vi "ni579x Send User Command.vi"(0 "Register Bus":T3, 1 "scope":string, 5 "User Command":T1 {"User Command ID" items=["Set Clock Select"=0, "Set CLK OUT Source"=1, "DAC Sync User Start"=2, "DAC Sync User End"=3, "Enable Baseband Amp"=5, "Set Rx Attenuation Pre-LNA"=7, "Set Rx Attenuation Post-LNA"=8, "Set Tx Attenuation"=9, "Set LO Filter"=32, "Set Front End Filter"=33, "Enable LO"=34, "Set Routing Mux"=37, "Read Current Rev Lower"=240, "Read Current Rev Upper"=241, "Read Oldest Compat Rev Lower"=242, "Read Oldest Compat Rev Upper"=243, "Re-Initialize"=255]; "User Data 1" format="%x"; "User Data 0" format="%x"}, 9 "timeout":dbl=1.0, 11 "Error In":errorcluster, 12 "wait for completion?":bool=TRUE, 13 "read return values?":bool=TRUE) -> (4 "Register Bus (out)":T3, 6 "user command status":u8, 8 "user return value":u16, 10 "user command error":u8, 15 "Error Out":errorcluster)   [LabVIEW 2015, in "ni579x Config v2 Host.lvlib"]
uses:
  <instrlib>/ni579x/Config/v2/Host/ni579x Config v2 Host.lvlib
  <instrlib>/_niInstr/Register Bus/v0/Host/Public/Register Bus Session.ctl
  <instrlib>/_niInstr/Register Bus/v0/Host/Private/Session Data.ctl
  <instrlib>/ni579x/Config/v2/Shared/Types/ni579x User Command.ctl
  <instrlib>/ni579x/Config/v2/Shared/Types/ni579x User Command ID.ctl
  <instrlib>/ni579x/Config/v2/Shared/Types/ni579x Register Bus Subsystem ID.ctl
  <instrlib>/_niInstr/Register Bus/v0/Host/Public/Register Write.ctl
  <instrlib>/_niInstr/Register Bus/v0/Host/Public/Register Read Request.ctl
  <instrlib>/ni579x/Config/v2/Shared/ni579x Config v2 Shared.lvlib
  <instrlib>/_niInstr/Register Bus/v0/Host/niInstr Register Bus v0 Host.lvlib
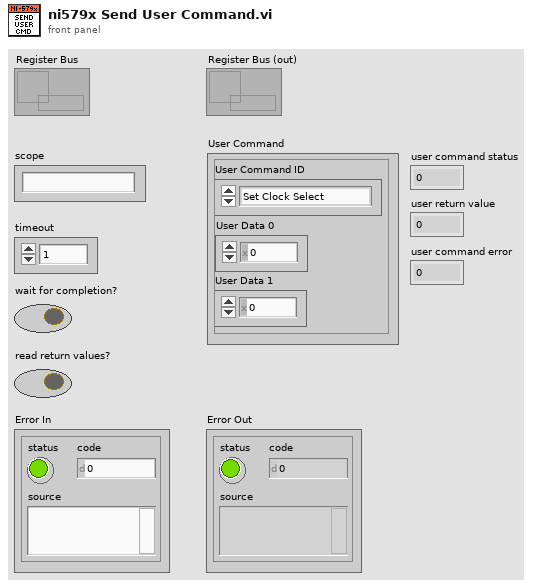
[diagram p1: front panel]
types:
  T1 = typedef "ni579x Config v2 Shared.lvlib/ni579x User Command.ctl" = cluster{"User Data 0":u8, "User Data 1":u8, "User Command ID":T2}
  T2 = typedef "ni579x Config v2 Shared.lvlib/ni579x User Command ID.ctl" = u8
  T3 = typedef "niInstr Register Bus v0 Host.lvlib/Register Bus Session.ctl" = refnum<queue>
  T4 = typedef "niInstr Register Bus v0 Host.lvlib/Register Write.ctl" = cluster{"subsystem":u8, "address":u16, "data":u32}
  T5 = typedef "niInstr Register Bus v0 Host.lvlib/Register Read Request.ctl" = cluster{"subsystem":u8, "address":u16}
  T6 = typedef "ni579x Config v2 Shared.lvlib/ni579x Register Bus Subsystem ID.ctl" = u8
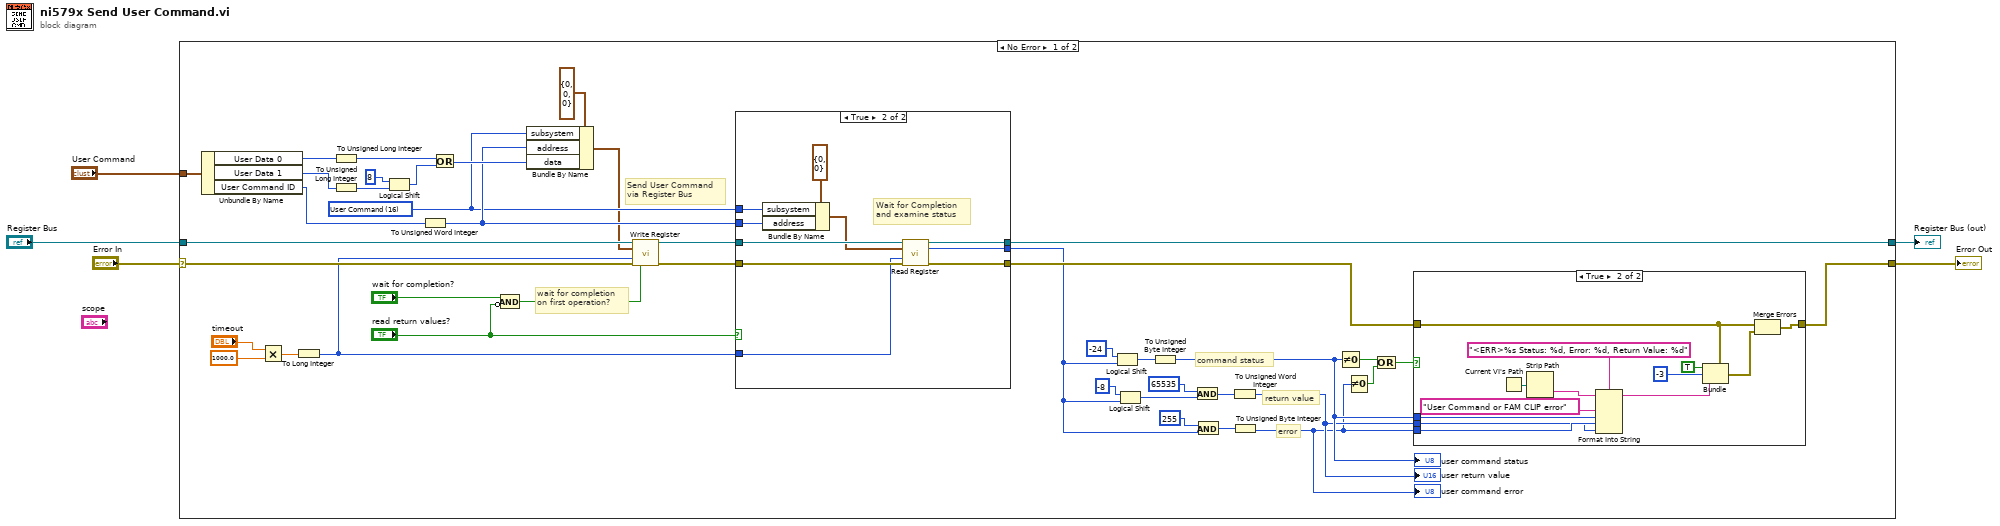
[diagram p0: block diagram]
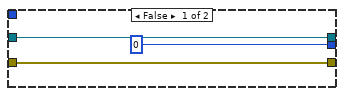
[diagram p2: hidden frame]
diagram:
  n1 = case shown="No Error" "Error In" {
    selector: "Error In" -> [w38 w76]
    tunnel: [w47 w76] -> w4
    tunnel: "Register Bus" -> [w37 w75]
    tunnel: "User Command" -> [w36 _]
    tunnel: [w20 w75] -> w1
    frame No Error {
      w8 = T6 16 items=["FAM Register Operation"=0, "User Command"=16, "Synchronization"=32] ("Subsystem ID")
      # "wait for completion \non first operation?"
      # "Send User Command \nvia Register Bus"
      # "error"
      # "return value"
      # "command status"
      n2 = Unbundle By Name(w36) -> ("User Data 0"=w35:u8, "User Data 1"=w34:u8, "User Command ID"=w33:T2)
      n3 = Multiply(x="timeout", y=1000.0) -> (x*y=w17:dbl)
      n4 = To Long Integer(number=w17) -> (32bit integer=w16:i32)
      n5 = To Unsigned Long Integer(number=w35) -> (unsigned 32bit integer=w43:u32)
      n6 = To Unsigned Long Integer(number=w34) -> (unsigned 32bit integer=w46:u32)
      n7 = Logical Shift(y=i8 8, x=w46) -> (x << y=w44:u32)
      n8 = To Unsigned Word Integer(number=w33) -> (unsigned 16bit integer=w40:u16)
      n9 = Or(x=w43, y=w44) -> (x .or. y?=w42:u32)
      n10 = Compound Arithmetic op=AND("wait for completion?", invert "read return values?") -> (w9:bool)
      n11 = Bundle By Name(cluster=T4 {"subsystem"=0, "address"=0, "data"=0} ("register write"), "subsystem"=w8, "address"=w40, "data"=w42) -> (w6:T4)
      n12 = call <instrlib>:"Write Register.vi"("session in"=w37, "register write"=w6, "timeout (1000 ms)"=w16, "error in"=w38, "wait until committed"=w9) -> ("session out"=w39:T3, "error out"=w41:errorcluster)  [unwired: 9 in]
      n13 = case shown="True" "read return values?" {
        tunnel: w41 -> [w50 w60]
        tunnel: w40 -> [_ w59]
        tunnel: w39 -> [w49 w58]
        tunnel: [w50 w57] -> w32
        tunnel: [u32 0 ("data") w56] -> w23
        tunnel: [w49 w55] -> w20
        tunnel: w8 -> [_ w52]
        tunnel: w16 -> [_ w51]
        frame False {
        }
        frame True {
          # "Wait for Completion \nand examine status"
          n14 = Bundle By Name(cluster=T5 {"subsystem"=0, "address"=0} ("register read request"), "subsystem"=w52, "address"=w59) -> (w53:T5)
          n15 = call <instrlib>:"Read Register.vi"("session in"=w58, "register read request"=w53, "timeout (1000 ms)"=w51, "error in"=w60) -> ("session out"=w55:T3, "data"=w56:u32, "error out"=w57:errorcluster)  [unwired: 9 in]
        }
      }
      n16 = Logical Shift(y=i8 -24, x=w23) -> (x << y=w30:u32)
      n17 = Logical Shift(y=i8 -8, x=w23) -> (x << y=w28:u32)
      n18 = To Unsigned Byte Integer(number=w30) -> (unsigned 8bit integer=w22:u8)
      "user command status" <- w22
      n19 = And(x=u32 65535, y=w28) -> (x .and. y?=w25:u32)
      n20 = And(x=u32 255, y=w23) -> (x .and. y?=w24:u32)
      n21 = To Unsigned Word Integer(number=w25) -> (unsigned 16bit integer=w21:u16)
      "user return value" <- w21
      n22 = To Unsigned Byte Integer(number=w24) -> (unsigned 8bit integer=w15:u8)
      "user command error" <- w15
      n23 = Not Equal To 0?(x=w22) -> (x != 0?=w14:bool)
      n24 = Not Equal To 0?(x=w15) -> (x != 0?=w13:bool)
      n25 = Or(x=w14, y=w13) -> (x .or. y?=w12:bool)
      n26 = case shown="True" w12 {
        tunnel: w32 -> [w61 w70]
        tunnel: [w61 w65] -> w47
        tunnel: w22 -> [_ w64]
        tunnel: w21 -> [_ w62]
        tunnel: w15 -> [_ w63]
        frame False {
        }
        frame True {
          n27 = Current VI's Path() -> (path=w73:path)
          n28 = Strip Path(path=w73) -> (name=w72:string)  [unwired: 1 out]
          n29 = Format Into String(format string="<ERR>%s Status: %d, Error: %d, Return Value: %d", initial string=w72, "User Command or FAM CLIP error" ("input 1"), w64, w63, w62) -> (resulting string=w71:string)  [unwired: 1 in, 1 out]
          n30 = Bundle(cluster=w70, "status"=TRUE, "code"=-3, "source"=w71) -> (w69:errorcluster)
          n31 = Merge Errors(w70, w69) -> (w65:errorcluster)
        }
      }
    }
    frame Error {
    }
  }
  "Error Out" <- w4
  "Register Bus (out)" <- w1
